vi "STICK_get_ports.vi"(5 "error in (no error)":errorcluster, 6 "VISA Refnum in":refnum<visa-resource-name>) -> (0 "error out":errorcluster, 1 "VISA Refnum out":refnum<visa-resource-name>, 2 "P2":T1, 3 "P1":T2, 4 "data":u8)   [LabVIEW 2014]
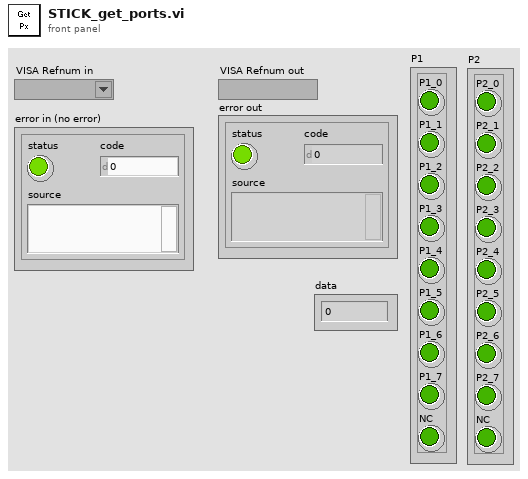
[diagram p1: front panel]
types:
  T1 = cluster{"P2_0":bool, "P2_1":bool, "P2_2":bool, "P2_3":bool, "P2_4":bool, "P2_5":bool, "P2_6":bool, "P2_7":bool, "NC":bool}
  T2 = cluster{"P1_0":bool, "P1_1":bool, "P1_2":bool, "P1_3":bool, "P1_4":bool, "P1_5":bool, "P1_6":bool, "P1_7":bool, "NC":bool}
  T3 = cluster{"Boolean array[0]":bool, "Boolean array[1]":bool, "Boolean array[2]":bool, "Boolean array[3]":bool, "Boolean array[4]":bool, "Boolean array[5]":bool, "Boolean array[6]":bool, "Boolean array[7]":bool, "Boolean array[8]":bool}
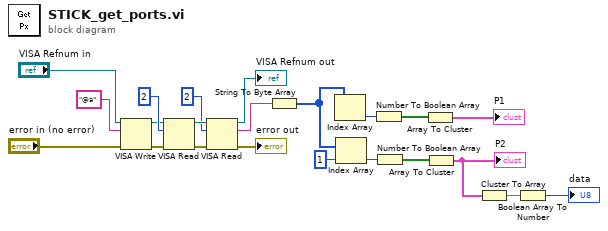
[diagram p0: block diagram]
diagram:
  n1 = VISA Write(VISA resource name="VISA Refnum in", write buffer="@a", error in (no error)="error in (no error)") -> (VISA resource name out=w19:refnum<visa-resource-name>, error out=w20:errorcluster)  [unwired: 1 out]
  n2 = VISA Read(VISA resource name=w19, byte count=u32 2, error in (no error)=w20) -> (VISA resource name out=w12:refnum<visa-resource-name>, error out=w13:errorcluster)  [unwired: 2 out]
  n3 = VISA Read(VISA resource name=w12, byte count=u32 2, error in (no error)=w13) -> (VISA resource name out=→"VISA Refnum out":refnum<visa-resource-name>, read buffer=w16:string, error out=→"error out":errorcluster)  [unwired: 1 out]
  n4 = String To Byte Array(string=w16) -> (unsigned byte array=w8:u8[])
  n5 = Index Array(array=w8) -> (element=w10:u8)  [unwired: 1 in]
  n6 = Index Array(array=w8, index=1) -> (element=w9:u8)
  n7 = Number To Boolean Array(number=w10) -> (Boolean array=w6:bool[])
  n8 = Number To Boolean Array(number=w9) -> (Boolean array=w5:bool[])
  n9 = Array To Cluster(array=w6) -> (cluster=→"P1":T3)
  n10 = Array To Cluster(array=w5) -> (cluster=w3:T3)
  "P2" <- w3
  n11 = Cluster To Array(cluster=w3) -> (array=w2:bool[])
  n12 = Boolean Array To Number(Boolean array=w2) -> (number=→"data":u32)
